vi "test.Variant.vi"(8 "error in":errorcluster, 10 "Data":variant, 11 "Command":string) -> (0 "error out":errorcluster, 3 "Return Data":variant)   [LabVIEW 2014]
uses:
  Private/Class/meth.Constructor.vi
  Private/Class/meth.Destructor.vi
  GLue.lvlib
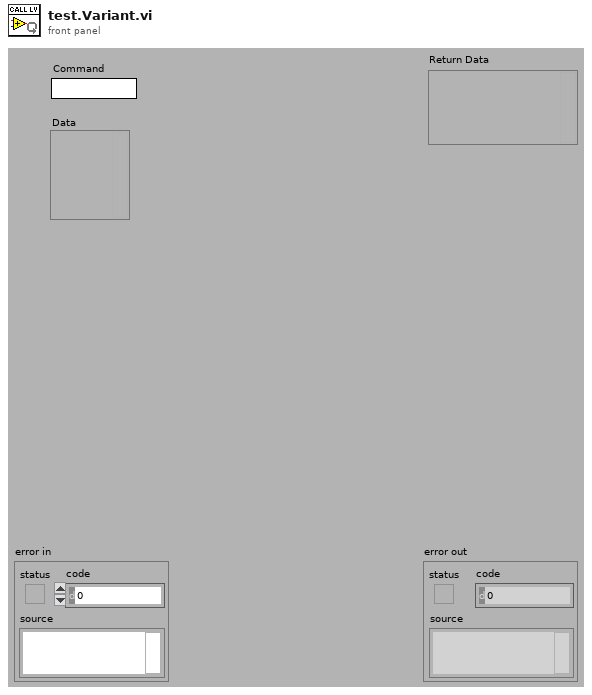
[diagram p1: front panel]
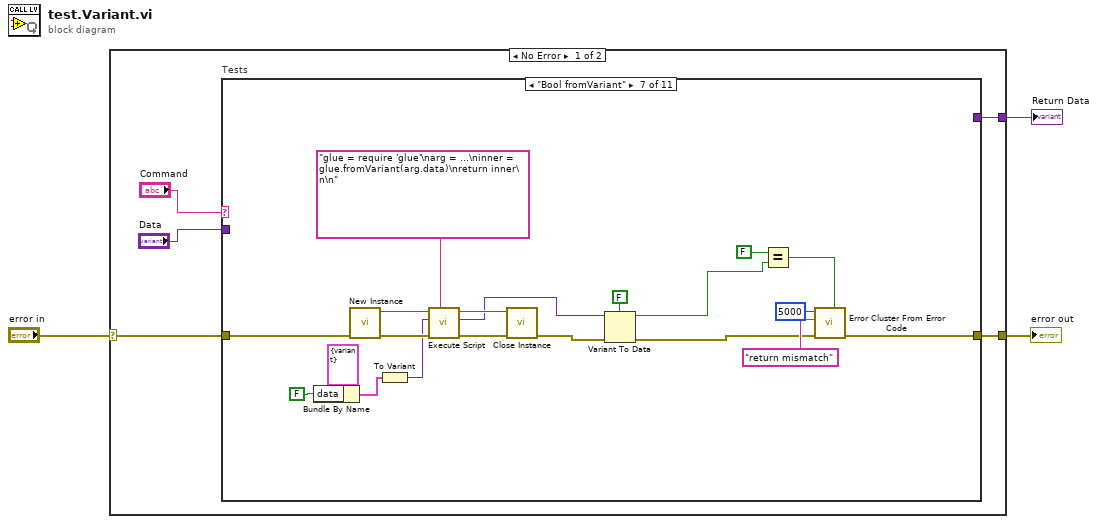
[diagram p0: block diagram]
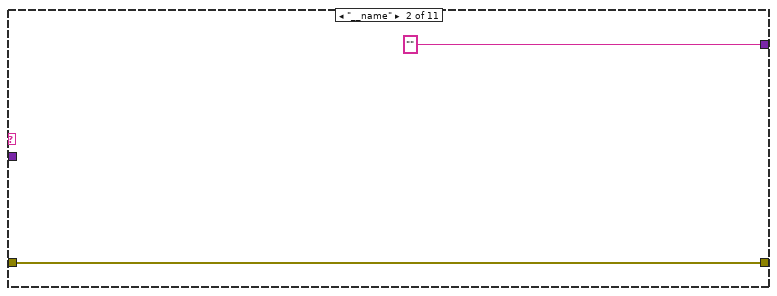
[diagram p3: hidden frame]
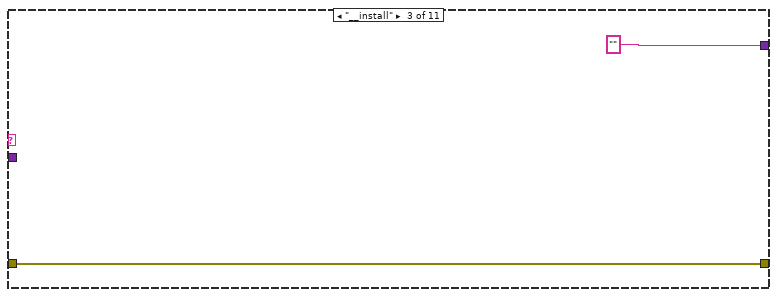
[diagram p4: hidden frame]
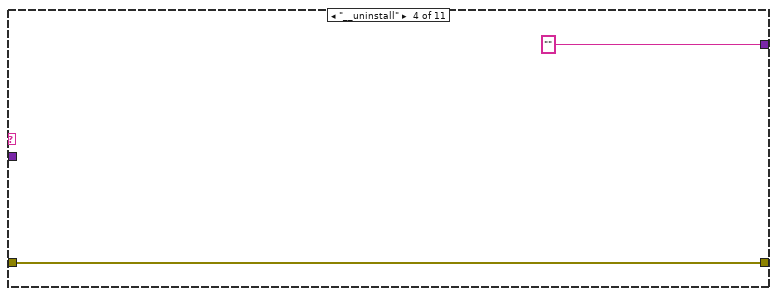
[diagram p5: hidden frame]
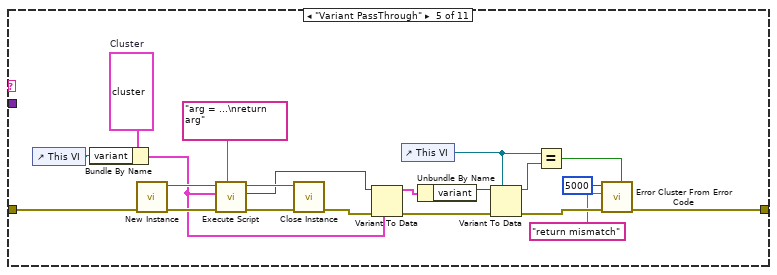
[diagram p6: hidden frame]
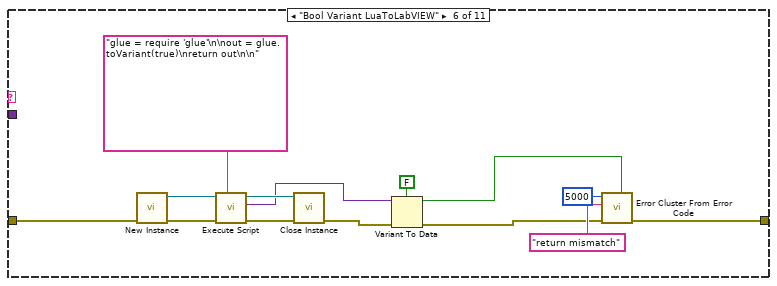
[diagram p7: hidden frame]
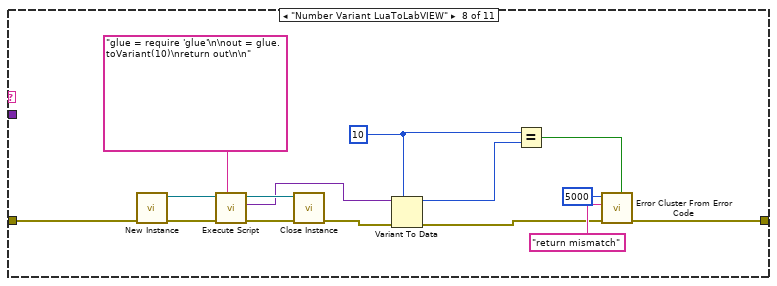
[diagram p8: hidden frame]
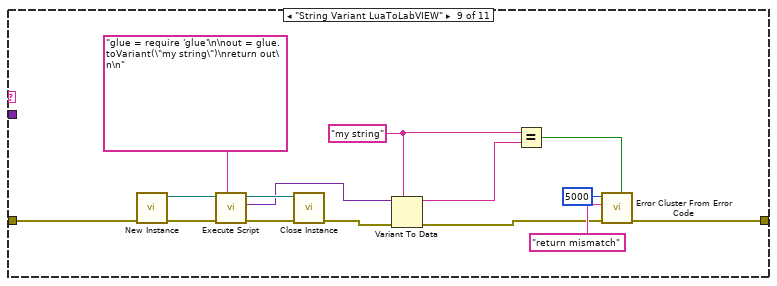
[diagram p9: hidden frame]
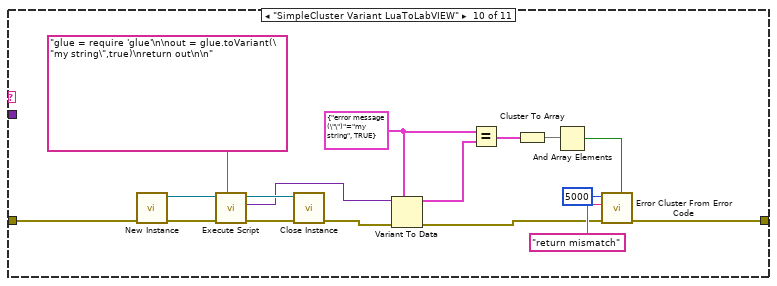
[diagram p10: hidden frame]
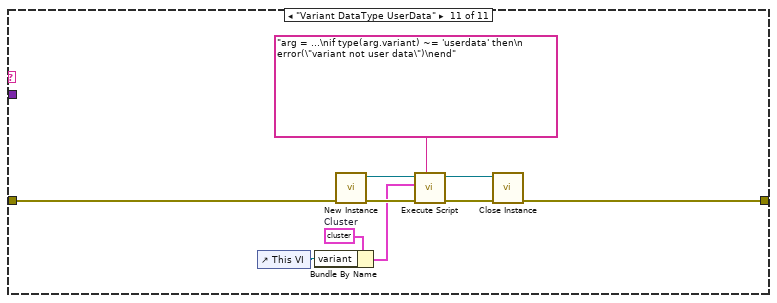
[diagram p11: hidden frame]
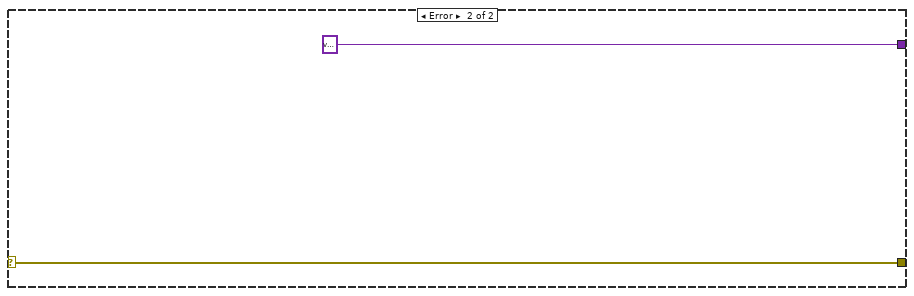
[diagram p12: hidden frame]
diagram:
  n1 = case shown="No Error" "error in" {
    selector: "error in" -> [w8 w130]
    tunnel: [w6 w130] -> w2
    tunnel: [w7 variant ("User Data")] -> w1
    frame No Error {
      n2 = case "Tests" shown="\"Bool fromVariant\"" "Command" {
        tunnel: w8 -> [w10 w11 w13 w15 w32 w46 w66 w81 w96 w113 w123]
        tunnel: "Data" -> [w9 _ _ _ _ _ _ _ _ _ _]
        tunnel: [w9 "" "" "" _ _ _ _ _ _ _] -> w7
        tunnel: [w10 w11 w13 w15 w20 w45 w65 w80 w95 w112 w119] -> w6
        frame Default {
        }
        frame "__name" {
        }
        frame "__install" {
        }
        frame "__uninstall" {
        }
        frame "Variant PassThrough" {
          w31 = cluster{"variant":variant, "temp":string} {"variant"=variant, "temp"=""}  # Cluster
          n3 = control-ref of="This VI"() -> (w30:refnum<vi>)
          n4 = Bundle By Name(cluster=w31, "variant"=w30) -> (w27:cluster{"variant":variant, "temp":string})
          n5 = call "New Instance.vi"("error in"=w32) -> ("error out"=w33:errorcluster, "GLue out"=w34:refnum<class "class.GLue.lvclass">)  [unwired: 9 in]
          n6 = call "Execute Script.vi"("Script"="arg = ...\nreturn arg", "error in"=w33, "Argument Data"=w27, "GLue in"=w34) -> ("error out"=w35:errorcluster, "Return Data"=w28:variant, "GLue out"=w36:refnum<class "class.GLue.lvclass">)  [unwired: 5 in]
          n7 = call "Close Instance.vi"("error in"=w35, "GLue in"=w36) -> ("error out"=w29:errorcluster)  [unwired: 9 in]
          n8 = Variant To Data(error in=w29, type=w27, Variant=w28) -> (data=w26:cluster{"variant":variant, "temp":string}, error out=w25:errorcluster)
          n9 = control-ref of="This VI"() -> (w23:refnum<vi>)
          n10 = Unbundle By Name(w26) -> ("variant"=w24:variant)
          n11 = Variant To Data(error in=w25, type=w23, Variant=w24) -> (data=w22:refnum<vi>, error out=w21:errorcluster)
          n12 = Equal?(x=w23, y=w22) -> (x = y?=w19:bool)
          n13 = call <vilib>:"Error Cluster From Error Code.vi"("is warning? (False)"=w19, "error in (no error)"=w21, "error message (\"\")"="return mismatch" ("error message (\"\")"), "error code (0)"=5000) -> ("error out"=w20:errorcluster)  [unwired: 5 in]
        }
        frame "Bool Variant LuaToLabVIEW" {
          n14 = call "New Instance.vi"("error in"=w46) -> ("error out"=w47:errorcluster, "GLue out"=w48:refnum<class "class.GLue.lvclass">)  [unwired: 9 in]
          n15 = call "Execute Script.vi"("Script"="glue = require 'glue'\n\nout = glue.toVariant(true)\nreturn out\n\n", "error in"=w47, "GLue in"=w48) -> ("error out"=w49:errorcluster, "Return Data"=w40:variant, "GLue out"=w50:refnum<class "class.GLue.lvclass">)  [unwired: 6 in]
          n16 = call "Close Instance.vi"("error in"=w49, "GLue in"=w50) -> ("error out"=w42:errorcluster)  [unwired: 9 in]
          n17 = Variant To Data(error in=w42, type=FALSE, Variant=w40) -> (data=w38:bool, error out=w41:errorcluster)
          n18 = call <vilib>:"Error Cluster From Error Code.vi"("is warning? (False)"=w38, "error in (no error)"=w41, "error message (\"\")"="return mismatch" ("error message (\"\")"), "error code (0)"=5000) -> ("error out"=w45:errorcluster)  [unwired: 5 in]
        }
        frame "Bool fromVariant" {
          n19 = Bundle By Name(cluster=cluster{"data":variant} {"data"=variant}, "data"=FALSE) -> (w56:cluster{"data":variant})
          n20 = call "New Instance.vi"("error in"=w66) -> ("error out"=w67:errorcluster, "GLue out"=w68:refnum<class "class.GLue.lvclass">)  [unwired: 9 in]
          n21 = To Variant(anything=w56) -> (Variant=w55:variant)
          n22 = call "Execute Script.vi"("Script"="glue = require 'glue'\narg = ...\ninner = glue.fromVariant(arg.data)\nreturn inner\n\n", "error in"=w67, "Argument Data"=w55, "GLue in"=w68) -> ("error out"=w69:errorcluster, "Return Data"=w57:variant, "GLue out"=w70:refnum<class "class.GLue.lvclass">)  [unwired: 5 in]
          n23 = call "Close Instance.vi"("error in"=w69, "GLue in"=w70) -> ("error out"=w62:errorcluster)  [unwired: 9 in]
          n24 = Variant To Data(error in=w62, type=FALSE, Variant=w57) -> (data=w53:bool, error out=w61:errorcluster)
          n25 = Equal?(x=FALSE, y=w53) -> (x = y?=w52:bool)
          n26 = call <vilib>:"Error Cluster From Error Code.vi"("is warning? (False)"=w52, "error in (no error)"=w61, "error message (\"\")"="return mismatch" ("error message (\"\")"), "error code (0)"=5000) -> ("error out"=w65:errorcluster)  [unwired: 5 in]
        }
        frame "Number Variant LuaToLabVIEW" {
          w74 = 10
          n27 = call "New Instance.vi"("error in"=w81) -> ("error out"=w82:errorcluster, "GLue out"=w83:refnum<class "class.GLue.lvclass">)  [unwired: 9 in]
          n28 = call "Execute Script.vi"("Script"="glue = require 'glue'\n\nout = glue.toVariant(10)\nreturn out\n\n", "error in"=w82, "GLue in"=w83) -> ("error out"=w84:errorcluster, "Return Data"=w75:variant, "GLue out"=w85:refnum<class "class.GLue.lvclass">)  [unwired: 6 in]
          n29 = call "Close Instance.vi"("error in"=w84, "GLue in"=w85) -> ("error out"=w77:errorcluster)  [unwired: 9 in]
          n30 = Variant To Data(error in=w77, type=w74, Variant=w75) -> (data=w73:i32, error out=w76:errorcluster)
          n31 = Equal?(x=w74, y=w73) -> (x = y?=w72:bool)
          n32 = call <vilib>:"Error Cluster From Error Code.vi"("is warning? (False)"=w72, "error in (no error)"=w76, "error message (\"\")"="return mismatch" ("error message (\"\")"), "error code (0)"=5000) -> ("error out"=w80:errorcluster)  [unwired: 5 in]
        }
        frame "String Variant LuaToLabVIEW" {
          w87 = "my string" ("error message (\"\")")
          n33 = call "New Instance.vi"("error in"=w96) -> ("error out"=w97:errorcluster, "GLue out"=w98:refnum<class "class.GLue.lvclass">)  [unwired: 9 in]
          n34 = call "Execute Script.vi"("Script"="glue = require 'glue'\n\nout = glue.toVariant(\"my string\")\nreturn out\n\n", "error in"=w97, "GLue in"=w98) -> ("error out"=w99:errorcluster, "Return Data"=w90:variant, "GLue out"=w100:refnum<class "class.GLue.lvclass">)  [unwired: 6 in]
          n35 = call "Close Instance.vi"("error in"=w99, "GLue in"=w100) -> ("error out"=w92:errorcluster)  [unwired: 9 in]
          n36 = Variant To Data(error in=w92, type=w87, Variant=w90) -> (data=w89:string, error out=w91:errorcluster)
          n37 = Equal?(x=w87, y=w89) -> (x = y?=w88:bool)
          n38 = call <vilib>:"Error Cluster From Error Code.vi"("is warning? (False)"=w88, "error in (no error)"=w91, "error message (\"\")"="return mismatch" ("error message (\"\")"), "error code (0)"=5000) -> ("error out"=w95:errorcluster)  [unwired: 5 in]
        }
        frame "SimpleCluster Variant LuaToLabVIEW" {
          w105 = cluster{"error message (\"\")":string, bool} {"error message (\"\")"="my string", TRUE}
          n39 = call "New Instance.vi"("error in"=w113) -> ("error out"=w114:errorcluster, "GLue out"=w115:refnum<class "class.GLue.lvclass">)  [unwired: 9 in]
          n40 = call "Execute Script.vi"("Script"="glue = require 'glue'\n\nout = glue.toVariant(\"my string\",true)\nreturn out\n\n", "error in"=w114, "GLue in"=w115) -> ("error out"=w116:errorcluster, "Return Data"=w107:variant, "GLue out"=w117:refnum<class "class.GLue.lvclass">)  [unwired: 6 in]
          n41 = call "Close Instance.vi"("error in"=w116, "GLue in"=w117) -> ("error out"=w109:errorcluster)  [unwired: 9 in]
          n42 = Variant To Data(error in=w109, type=w105, Variant=w107) -> (data=w106:cluster{"error message (\"\")":string, bool}, error out=w108:errorcluster)
          n43 = Equal?(x=w105, y=w106) -> (x = y?=w103:cluster{"error message (\"\")":bool, bool})
          n44 = Cluster To Array(cluster=w103) -> (array=w102:bool[])
          n45 = And Array Elements(Boolean array=w102) -> (logical AND=w104:bool)
          n46 = call <vilib>:"Error Cluster From Error Code.vi"("is warning? (False)"=w104, "error in (no error)"=w108, "error message (\"\")"="return mismatch" ("error message (\"\")"), "error code (0)"=5000) -> ("error out"=w112:errorcluster)  [unwired: 5 in]
        }
        frame "Variant DataType UserData" {
          w122 = cluster{"variant":variant, "temp":string} {"variant"=variant, "temp"=""}  # Cluster
          n47 = control-ref of="This VI"() -> (w121:refnum<vi>)
          n48 = Bundle By Name(cluster=w122, "variant"=w121) -> (w120:cluster{"variant":variant, "temp":string})
          n49 = call "New Instance.vi"("error in"=w123) -> ("error out"=w124:errorcluster, "GLue out"=w125:refnum<class "class.GLue.lvclass">)  [unwired: 9 in]
          n50 = call "Execute Script.vi"("Script"="arg = ...\nif type(arg.variant) ~= 'userdata' then\n error(\"variant not user data\")\nend", "error in"=w124, "Argument Data"=w120, "GLue in"=w125) -> ("error out"=w126:errorcluster, "GLue out"=w127:refnum<class "class.GLue.lvclass">)  [unwired: 5 in, 1 out]
          n51 = call "Close Instance.vi"("error in"=w126, "GLue in"=w127) -> ("error out"=w119:errorcluster)  [unwired: 9 in]
        }
      }
    }
    frame Error {
    }
  }
  "Return Data" <- w1
  "error out" <- w2
